vi "pessimize_err_fun.vi"(10 "Pessimize fun info":T1 {"Point selector"."Light number" min=0 max=5}, 11 "Error":dbl[](array[numeric])) -> (3 "Result":dbl)   [LabVIEW 2013]
uses:
  pessimize_objective_fun_info.ctl
  calibration/point_selector.ctl
  ui_override_opts.ctl
  <vilib>/Analysis/Matrix/Datatypes/RealMatrix.ctl
  <vilib>/Analysis/Matrix/NI_Matrix.lvlib
panel:
  # "Generate scalar result from pose error vector, according to scaling and criterion."
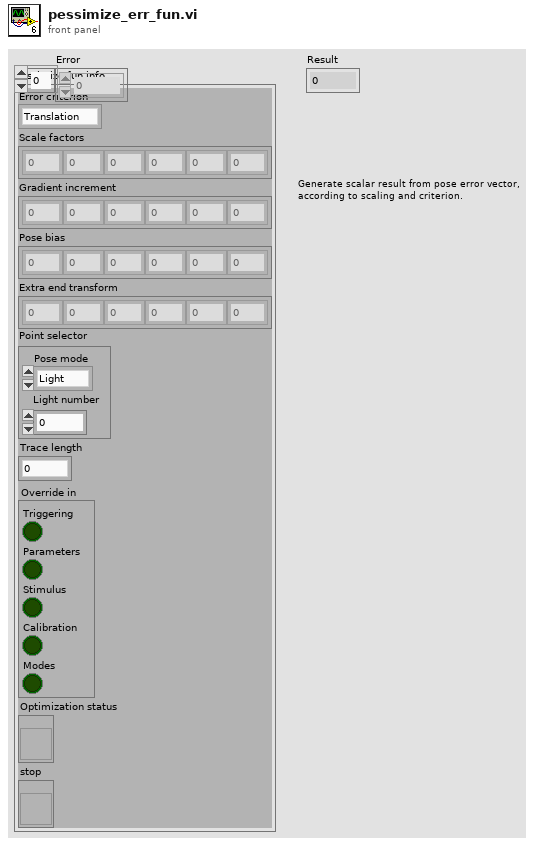
[diagram p1: front panel]
types:
  T1 = typedef "pessimize_objective_fun_info.ctl" = cluster{"Error criterion":enum16{"Translation", "Orientation", "Moment"}, "Scale factors":dbl[], "Gradient increment":dbl[], "Pose bias":dbl[], "Extra end transform":dbl[], "Point selector":T2, "Trace length":dbl, "Override in":T3, "Optimization status":refnum<vi>, "stop":refnum<vi>}
  T2 = typedef "point_selector.ctl" = cluster{"Pose mode":enum16{"Light", "Handle", "Output"}, "Light number":i32}
  T3 = typedef "ui_override_opts.ctl" = cluster{"Triggering":bool, "Parameters":bool, "Stimulus":bool, "Calibration":bool, "Modes":bool}
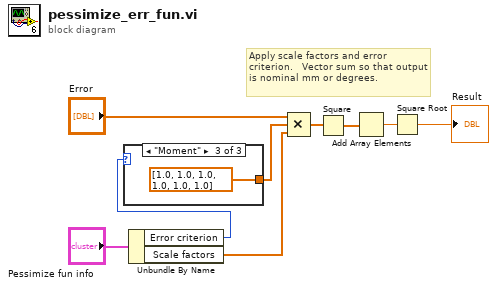
[diagram p0: block diagram]
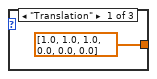
[diagram p2: hidden frame]
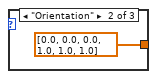
[diagram p3: hidden frame]
diagram:
  # "Apply scale factors and error criterion.   Vector sum so that output is nominal mm or degrees."
  n1 = Unbundle By Name("Pessimize fun info") -> ("Error criterion"=w9:enum16{"Translation", "Orientation", "Moment"}, "Scale factors"=w1:dbl[])
  n2 = case shown="\"Moment\"" w9 {
    tunnel: [dbl[] [1.0, 1.0, 1.0, 0.0, 0.0, 0.0] ("Scale factors") dbl[] [0.0, 0.0, 0.0, 1.0, 1.0, 1.0] ("Scale factors") dbl[] [1.0, 1.0, 1.0, 1.0, 1.0, 1.0] ("Scale factors")] -> w5
    frame "Translation" {
    }
    frame "Orientation" {
    }
    frame "Moment" {
    }
  }
  n3 = Compound Arithmetic op=MULTIPLY("Error", w5, w1) -> (w7:dbl[])
  n4 = Square(x=w7) -> (x^2=w6:dbl[])
  n5 = Add Array Elements(numeric array=w6) -> (sum=w3:dbl)
  n6 = Square Root(x=w3) -> (sqrt(x)=→"Result":dbl)
